vi "2D Chop One Bin.vi"(4 "tolerance":dbl=1e-16, 6 "VI ref":cluster{"f(X)":refnum<vi>, "data":variant}, 7 "Formula":T1, 8 "error in (no error)":errorcluster, 9 "Formula/VI ref":bool, 10 "chop x?":bool, 11 "Bins In":T3={"bin x"={"lower limit"=0.0, "upper limit"=1.0}, "bin y"={"lower limit"=0.0, "upper limit"=1.0}}) -> (0 "error out":errorcluster, 2 "Chop x Out":bool[](array[boolean]), 3 "Bins Out":T2(array[cluster]))   [LabVIEW 2014, in "NI_AALPro.lvlib"]
uses:
  NI_AALPro.lvlib
  A x Vector.vi
  Real Dot Product.vi
  NI_AALBase.lvlib
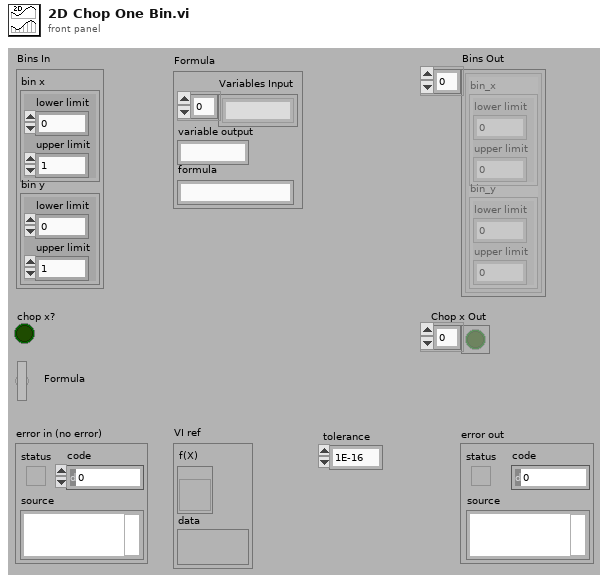
[diagram p1: front panel]
types:
  T1 = cluster{"Variables Input":string[], "variable output":string, "formula":string}
  T2 = cluster{"bin_x":cluster{"lower limit":dbl, "upper limit":dbl}, "bin_y":cluster{"lower limit":dbl, "upper limit":dbl}}[]
  T3 = cluster{"bin x":cluster{"lower limit":dbl, "upper limit":dbl}, "bin y":cluster{"lower limit":dbl, "upper limit":dbl}}
  T4 = cluster{"bin x":cluster{"lower limit":dbl, "upper limit":dbl}, "bin y":cluster{"lower limit":dbl, "upper limit":dbl}}[]
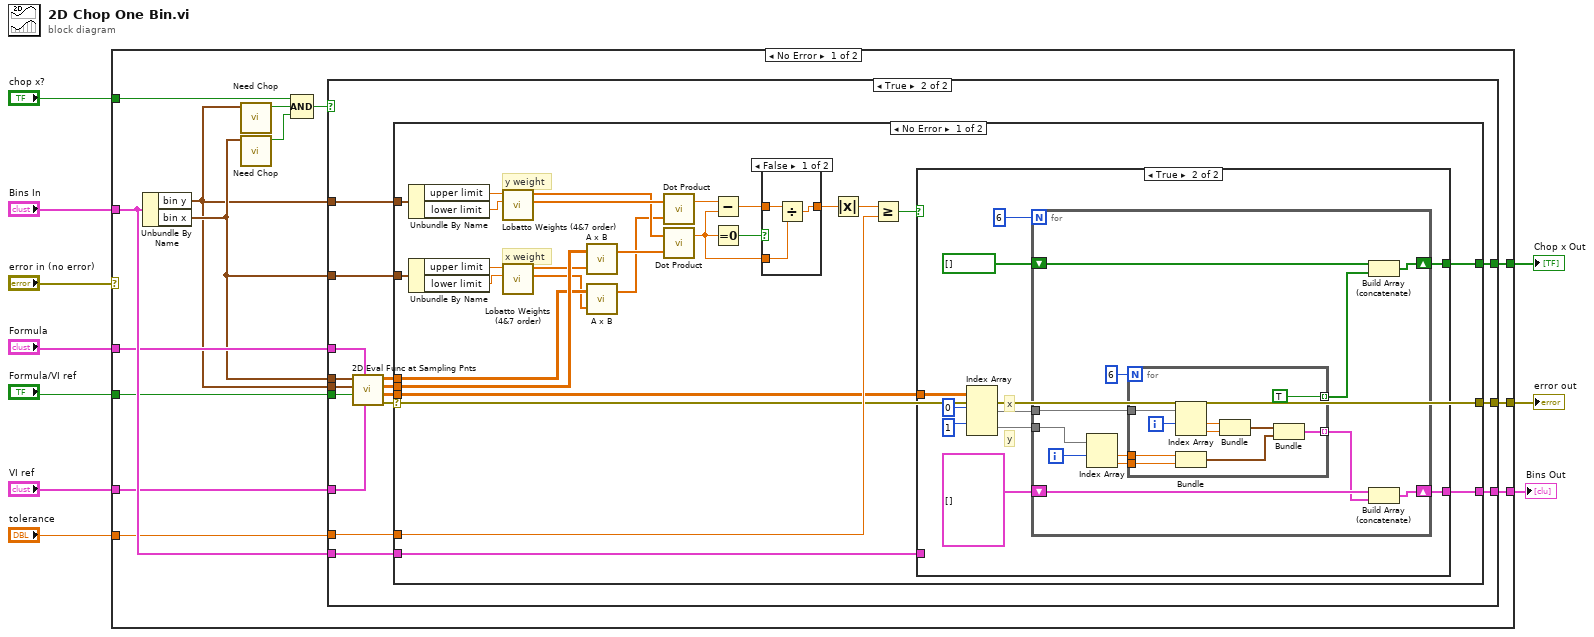
[diagram p0: block diagram]
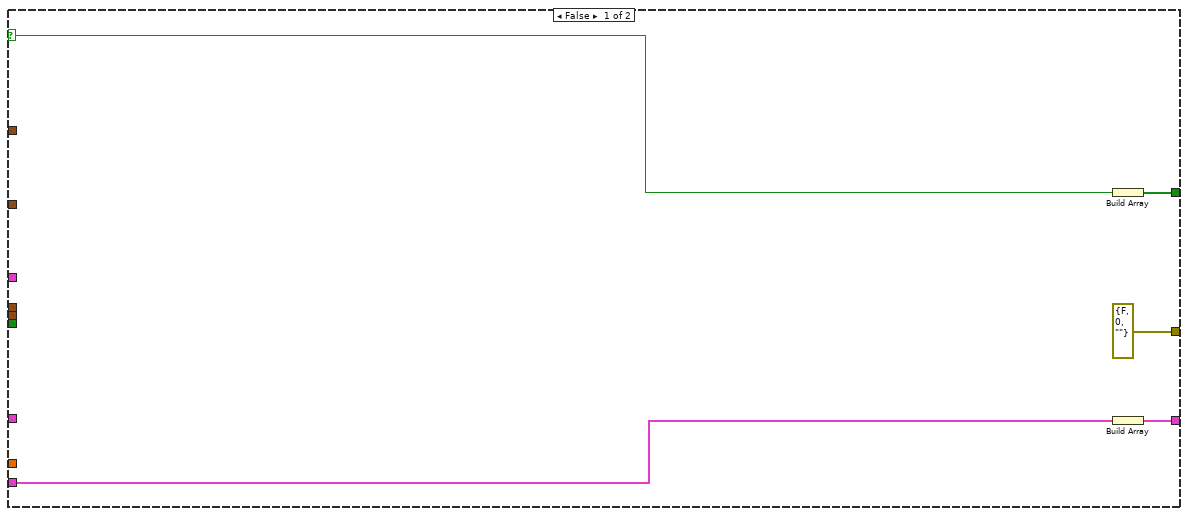
[diagram p2: hidden frame]
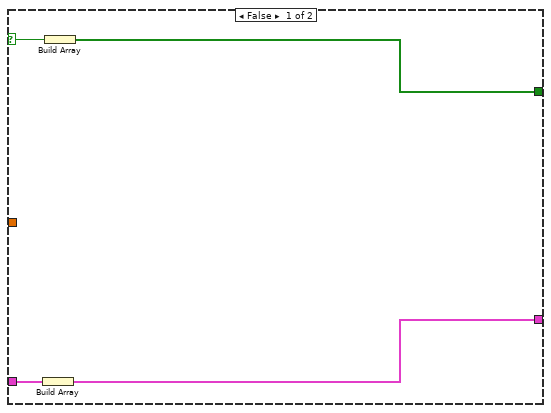
[diagram p4: hidden frame]
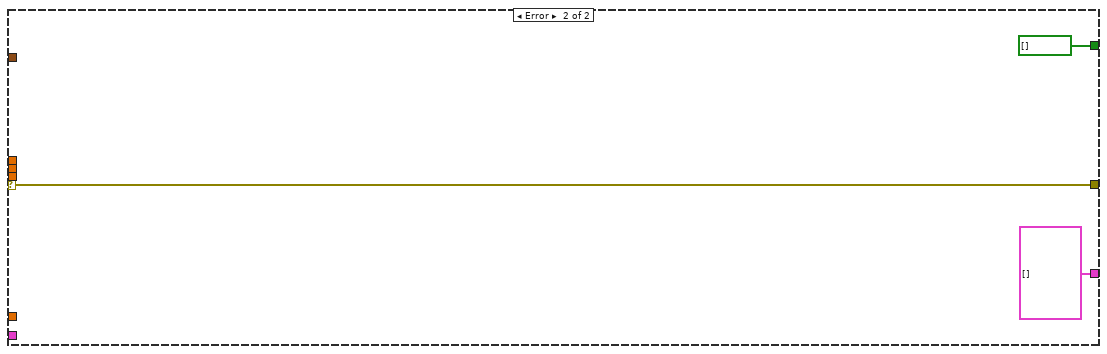
[diagram p5: hidden frame]
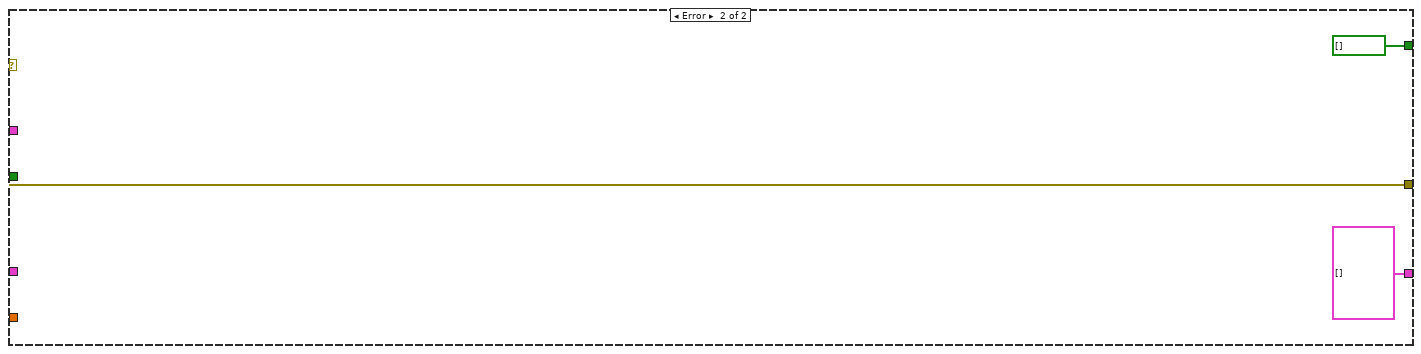
[diagram p6: hidden frame]
diagram:
  n1 = case shown="No Error" "error in (no error)" {
    selector: "error in (no error)" -> [_ w118]
    tunnel: "Bins In" -> [w24 _]
    tunnel: [w23 bool[] [] ("Chop x Out")] -> w9
    tunnel: "tolerance" -> [w22 _]
    tunnel: "chop x?" -> [w20 _]
    tunnel: [w19 T2 [] ("Bins Out")] -> w6
    tunnel: "Formula" -> [w18 _]
    tunnel: "Formula/VI ref" -> [w17 _]
    tunnel: "VI ref" -> [w16 _]
    tunnel: [w11 w118] -> w2
    frame No Error {
      n2 = Unbundle By Name(w24) -> ("bin y"=w12:cluster{"lower limit":dbl, "upper limit":dbl}, "bin x"=w13:cluster{"lower limit":dbl, "upper limit":dbl})
      n3 = call "Need Chop.vi"("bin"=w12) -> ("chop?"=w15:bool)  [unwired: 10 out]
      n4 = call "Need Chop.vi"("bin"=w13) -> ("chop?"=w14:bool)  [unwired: 10 out]
      n5 = Compound Arithmetic op=AND(w20, w15, w14) -> (w21:bool)
      n6 = case shown="True" w21 {
        selector: w21 -> [w29 _]
        tunnel: [w27 w45] -> w19
        tunnel: [w28 w44] -> w23
        tunnel: w22 -> [_ w43]
        tunnel: w16 -> [_ w41]
        tunnel: w13 -> [_ w40]
        tunnel: w12 -> [_ w39]
        tunnel: w24 -> [w26 w36]
        tunnel: w18 -> [_ w35]
        tunnel: w17 -> [_ w34]
        tunnel: w13 -> [_ w33]
        tunnel: w12 -> [_ w32]
        tunnel: [errorcluster {"status"=FALSE, "code"=0, "source"=""} ("error out") w30] -> w11
        frame False {
          n7 = Build Array(w29) -> (w28:bool[])
          n8 = Build Array(w26) -> (w27:T4)
        }
        frame True {
          n9 = call "2D Eval Func at Sampling Pnts.vi"("VI ref"=w41, "Formula"=w35, "Formula/VI ref"=w34, "y limit"=w39, "x limit"=w40) -> ("error out"=w31:errorcluster, "Sampling points (7-order)"=w38:dbl[][], "Function Evaluations (4 pts)"=w37:dbl[][], "Function Evaluations (7 pts)"=w42:dbl[][])  [unwired: 1 in, 2 out]
          n10 = case shown="No Error" w31 {
            selector: w31 -> [w52 w115]
            tunnel: [w71 T2 [] ("Bins Out")] -> w45
            tunnel: [w70 bool[] [] ("Chop x Out")] -> w44
            tunnel: w43 -> [w69 _]
            tunnel: w42 -> [w48 _]
            tunnel: w38 -> [w65 _]
            tunnel: w37 -> [w51 _]
            tunnel: w36 -> [w60 _]
            tunnel: w33 -> [w58 _]
            tunnel: w32 -> [w53 _]
            tunnel: [w52 w115] -> w30
            frame No Error {
              # "y weight"
              # "x weight"
              n11 = Unbundle By Name(w53) -> ("upper limit"=w55:dbl, "lower limit"=w54:dbl)
              n12 = Unbundle By Name(w58) -> ("upper limit"=w57:dbl, "lower limit"=w56:dbl)
              n13 = call "Lobatto Weights (4&7 order).vi"("lower limit"=w54, "upper limit"=w55) -> ("Weights (7-Order)"=w64:dbl[], "Weights (4-Order)"=w59:dbl[])  [unwired: 8 out]
              n14 = call "Lobatto Weights (4&7 order).vi"("lower limit"=w56, "upper limit"=w57) -> ("Weights (7-Order)"=w47:dbl[], "Weights (4-Order)"=w50:dbl[])  [unwired: 8 out]
              n15 = call-poly "A x B.vi"("Vector"=w50, "A"=w51) -> ("A x Vector"=w49:dbl[])  [unwired: 1 out]
              n16 = call-poly "A x B.vi"("Vector"=w47, "A"=w48) -> ("A x Vector"=w46:dbl[])  [unwired: 1 out]
              n17 = call-poly "Dot Product.vi"("Y Vector"=w46, "X Vector"=w64) -> ("X * Y"=w63:dbl)  [unwired: 1 out]
              n18 = call-poly "Dot Product.vi"("Y Vector"=w49, "X Vector"=w59) -> ("X * Y"=w62:dbl)  [unwired: 1 out]
              n19 = Subtract(x=w63, y=w62) -> (x-y=w67:dbl)
              n20 = Equal To 0?(x=w62) -> (x = 0?=w68:bool)
              n21 = case shown="False" w68 {
                tunnel: w67 -> [w75 w76]
                tunnel: w62 -> [w74 _]
                tunnel: [w73 w76] -> w66
                frame False {
                  n22 = Divide(x=w75, y=w74) -> (x/y=w73:dbl)
                }
                frame True {
                }
              }
              n23 = Absolute Value(x=w66) -> (abs(x)=w61:dbl)
              n24 = Greater Or Equal?(x=w61, y=w69) -> (x >= y?=w72:bool)
              n25 = case shown="True" w72 {
                selector: w72 -> [w78 _]
                tunnel: w65 -> [_ w90]
                tunnel: [w79 w81] -> w71
                tunnel: w60 -> [w80 _]
                tunnel: [w77 w83] -> w70
                frame False {
                  n26 = Build Array(w80) -> (w79:T4)
                  n27 = Build Array(w78) -> (w77:bool[])
                }
                frame True {
                  # "y"
                  # "x"
                  n28 = Index Array(array=w90, index (row) #1=0 ("index (row)"), index (row) #2=1 ("index (row)")) -> (element #1=w89:dbl[], element #2=w86:dbl[])  [unwired: 2 in]
                  n29 = for {
                    N: 6 -> [_]
                    tunnel: w89 -> [w101]
                    tunnel: w86 -> [w99]
                    shift-right: [w94] -> w83
                    shift-left: bool[] [] ("Chop x Out") -> [w95]
                    shift-right: [w91] -> w81
                    shift-left: T2 [] ("Bins Out") -> [w93]
                    i -> [w100]
                    n30 = Index Array(array=w99, index #1=w100) -> (element #1=w98:dbl, element #2=w97:dbl)  [unwired: 1 in]
                    n31 = for {
                      N: 6 -> [_]
                      tunnel: w101 -> [w112]
                      tunnel: [TRUE] -> w96 mode=indexing
                      tunnel: w98 -> [w107]
                      tunnel: w97 -> [w106]
                      tunnel: [w103] -> w92 mode=indexing
                      i -> [w111]
                      n32 = Index Array(array=w112, index #1=w111) -> (element #1=w109:dbl, element #2=w110:dbl)  [unwired: 1 in]
                      n33 = Bundle(w107, w106) -> (w104:cluster{dbl, dbl})  [unwired: 1 out]
                      n34 = Bundle(w109, w110) -> (w105:cluster{dbl, dbl})  [unwired: 1 out]
                      n35 = Bundle(w105, w104) -> (w103:cluster{cluster{dbl, dbl}, cluster{dbl, dbl}})  [unwired: 1 out]
                    }
                    n36 = Build Array (concatenate)(w95, w96) -> (w94:bool[])
                    n37 = Build Array (concatenate)(w93, w92) -> (w91:T2)
                  }
                }
              }
            }
            frame Error {
            }
          }
        }
      }
    }
    frame Error {
    }
  }
  "Chop x Out" <- w9
  "error out" <- w2
  "Bins Out" <- w6
